vi "Actor Core.vi"(8 "error in":errorcluster, 11 "DUALSCREEN in":refnum<class "DualScreenV.lvclass">) -> (0 "error out":errorcluster, 3 "Actor out":refnum<class "Actor.lvclass">)   [LabVIEW 2020, in "DualScreenV.lvlib" / "DualScreenV.lvclass"]
uses:
  DualScreenV.lvclass
  support/Actor Framework.lvlibp/1abvi3w/vi.lib/ActorFramework/Actor/Actor.lvclass
  support/UI_Actor.lvlibp/UI_Actor Messages/UI_Resize Msg/UI_Resize Msg.lvclass
  support/Actor Framework.lvlibp/1abvi3w/vi.lib/ActorFramework/Stop Msg/Stop Msg.lvclass
  D:/Projets/STEP AT/Bahamut/D&Cs/DualScreen/DualScreen/DualScreen.lvclass
  D:/Projets/STEP AT/Bahamut/D&Cs/D&C_SchemaBase/D&C_SchemaBase/D&C_SchemaBase.lvclass
  D:/Projets/STEP AT/Bahamut/support/UI_Actor.lvlibp/UI_Actor/UI_Actor.lvclass
  D:/Projets/STEP AT/Bahamut/support/Actor Framework.lvlibp/1abvi3w/vi.lib/ActorFramework/Actor/Actor.lvclass
  D:/Projets/STEP AT/Bahamut/D&Cs/DualScreenV/DualScreenV/DualScreenV.lvclass
  DualScreen/DualScreen/DualScreen.lvclass
panel:
  in  "DynStop":bool
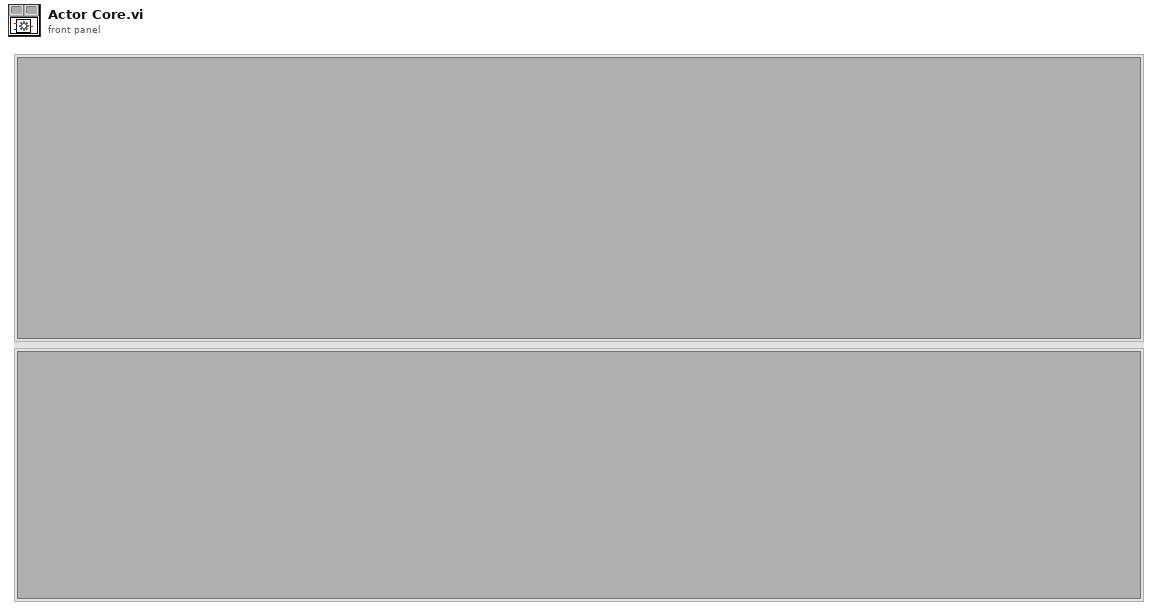
[diagram p1: front panel]
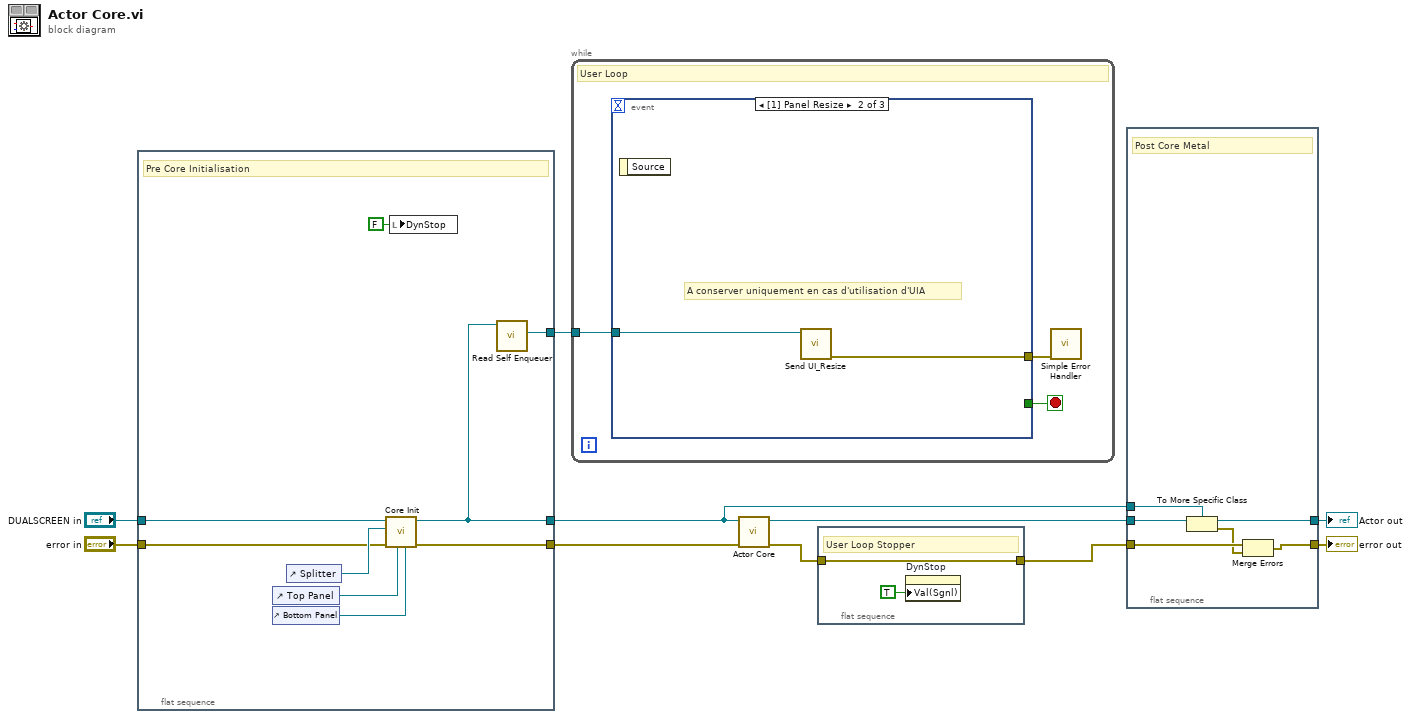
[diagram p0: block diagram]
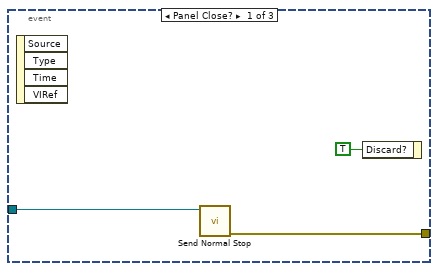
[diagram p2: hidden frame]
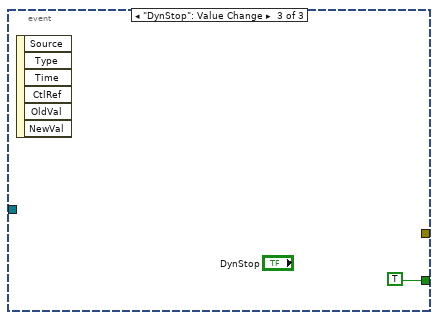
[diagram p3: hidden frame]
diagram:
  n1 = flat-sequence {
    tunnel: [w13] -> w4
    tunnel: "DUALSCREEN in" -> [w12]
    tunnel: [w11] -> w9
    tunnel: "error in" -> [w14]
    tunnel: [w18] -> w1
    frame #0 {
      # "Pre Core Initialisation"
      n2 = control-ref of="Top Panel"() -> (w16:refnum<vi>)
      n3 = control-ref of="Bottom Panel"() -> (w15:refnum<vi>)
      n4 = control-ref of="Splitter"() -> (w17:refnum<vi>)
      n5 = call "Core Init.vi"("2nd Panel"=w15, "1st Panel"=w16, "error in (no error)"=w14, "Splitter ref"=w17, "DualScreen in"=w12) -> ("error out"=w11:errorcluster, "DualScreen out"=w13:refnum<class "DualScreenV.lvclass">)  [unwired: 5 in]
      n6 = local write "DynStop"(FALSE ("DynStop")) -> ()
      n7 = call "Read Self Enqueuer.vi"("Actor"=w13) -> ("Self Enqueuer"=w18:refnum<class "Message Enqueuer.lvclass">)  [unwired: 10 in]
    }
  }
  n8 = while {
    tunnel: w1 -> [w21]
    stop <- w22 stop-if-true
    # "User Loop"
    n9 = event shown="[1] Panel Resize" {
      selector: _ -> [_ _ _]
      dyn-events: _ -> [_ _ _]
      timeout: _ -> [_ _ _]
      tunnel: [_ _ TRUE] -> w22
      tunnel: w21 -> [w24 w27 _]
      tunnel: [w23 w26 _] -> w20
      event Panel Close? {
        n10 = event-data() -> ()  [unwired: 1 in, 4 out]
        n11 = call "Send Normal Stop.vi"("Message Enqueuer"=w24) -> ("error out"=w23:errorcluster)  [unwired: 10 in]
        n12 = event-data("Discard?"=TRUE) -> ()  [unwired: 1 in, 1 out]
      }
      event Panel Resize {
        # "A conserver uniquement en cas d'utilisation d'UIA"
        n13 = event-data() -> ()  [unwired: 1 in, 1 out]
        n14 = call "Send UI_Resize.vi"("Message Enqueuer"=w27) -> ("error out"=w26:errorcluster)  [unwired: 9 in, 1 out]
      }
      event "DynStop": Value Change {
        n15 = event-data() -> ()  [unwired: 1 in, 6 out]
      }
    }
    n16 = call <vilib>:"Simple Error Handler.vi"("error in (no error)"=w20) -> ()  [unwired: 4 in, 5 out]
  }
  n17 = call-parent "Actor Core.vi"("error in"=w9, "UI_Actor in"=w4) -> ("error out"=w10:errorcluster, "Actor out"=w8:refnum<class "Actor.lvclass">)  [unwired: 8 in]
  n18 = flat-sequence {
    tunnel: [w29] -> w7
    tunnel: w10 -> [w29]
    frame #0 {
      # "User Loop Stopper"
      n19 = property on="DynStop" class="Bool (strict)"("Val(Sgnl)"=TRUE ("Value (Signaling)")) -> ()  [unwired: 2 in, 2 out]
    }
  }
  n20 = flat-sequence {
    tunnel: [w35] -> w3
    tunnel: w8 -> [w36]
    tunnel: w7 -> [w33]
    tunnel: w4 -> [w34]
    tunnel: [w31] -> w2
    frame #0 {
      # "Post Core Metal"
      n21 = To More Specific Class(target class=w34, reference=w36) -> (specific class reference=w35:refnum<class "DualScreenV.lvclass">, error out=w32:errorcluster)  [unwired: 1 in]
      n22 = Merge Errors(w33, w32) -> (w31:errorcluster)
    }
  }
  "error out" <- w2
  "Actor out" <- w3
